vi "Set parameter.vi"(8 "error in (no error)":errorcluster, 10 "Parameter":T1, 11 "Sensor General Class in":refnum<class "Sensor General Class.lvclass">) -> (0 "error out":errorcluster, 3 "Sensor General Class out":refnum<class "Sensor General Class.lvclass">)   [LabVIEW 2020, in "Sensor General Class.lvclass"]
uses:
  Sensor General Class.lvclass
  Parameters Enum.ctl
  Sensor General Class.lvclass/Sensor General Class.ctl
panel:
  in  "Data":u16[](array[numeric])
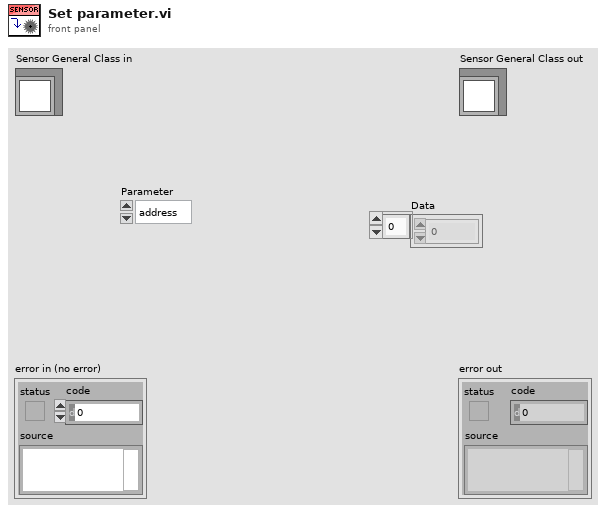
[diagram p1: front panel]
types:
  T1 = typedef "Sensor General Class.lvclass/Parameters Enum.ctl" = enum16{"address", "baud rate", "parity check", "load", "insulating gas", "additional component", "s/n", "hardware version", "firmware version", "humidity enable", "tag", "pressure offset", "humidity offset", "temperature offset", "service code"}
  T2 = cluster{"Mode":enum16{"RTU", "ASCII"}, "Slave Address":u8}
  T3 = cluster{"index":i32, "name":string, "register":u16, "word count":u16, "Write":bool}[]
  T4 = cluster{"index":i32, "name":string, "register":u16, "word count":u16, "Write":bool}
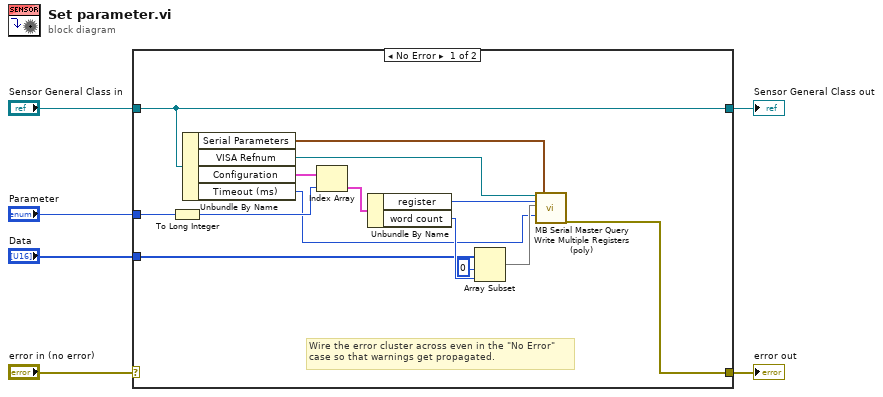
[diagram p0: block diagram]
diagram:
  n1 = case shown="No Error" "error in (no error)" {
    selector: "error in (no error)" -> [_ w22]
    tunnel: [w7 w22] -> w5
    tunnel: [w20 w21] -> w3
    tunnel: "Sensor General Class in" -> [w20 w21]
    tunnel: "Data" -> [w10 _]
    tunnel: "Parameter" -> [w17 _]
    frame No Error {
      # "Wire the error cluster across even in the \"No Error\"\ncase so that warnings get propagated."
      n2 = To Long Integer(number=w17) -> (32bit integer=w15:i32)
      n3 = Unbundle By Name(w20) -> ("Serial Parameters"=w19:T2, "VISA Refnum"=w18:refnum<visa-resource-name>, "Configuration"=w16:T3, "Timeout (ms)"=w8:u32)
      n4 = Index Array(array=w16, index=w15) -> (element=w14:T4)
      n5 = Unbundle By Name(w14) -> ("register"=w13:u16, "word count"=w12:u16)
      n6 = Array Subset(array=w10, index=0, length=w12) -> (w9:u16[])
      n7 = call <vilib>:"MB Serial Master Query Write Multiple Registers (poly).vi"("VISA resource name"=w18, "Starting Address"=w13, "Registers"=w9, "Timeout"=w8, "Serial Parameters"=w19) -> ("error out"=w7:errorcluster)  [unwired: 12 in, 2 out]
    }
    frame Error {
    }
  }
  "error out" <- w5
  "Sensor General Class out" <- w3
